vi "Auto - Values into Cluster (SubVI).vi"(6 "Auto Array":dbl[][](array[numeric]), 7 "Was Disabled":bool, 8 "Constant cluster In":T2, 9 "Auton Input Cluster in":T3, 10 "Sensors In":T1, 11 "Auton State":i32) -> (0 "Sensor TypeDef.ctlConstant cluster Out":T2, 1 "Auton Input Cluster With Data":T3, 2 "Sensors Out":T1, 3 "Auton State Out":i32)   [LabVIEW 2020]
uses:
  TypeDefs/Auton Cluster Typedef.ctl
  Disabled/Constant VI_s/Disabled - Constant Cluster Typedef.ctl
  TypeDefs/Sensor TypeDef.ctl
panel:
  # "Controls"
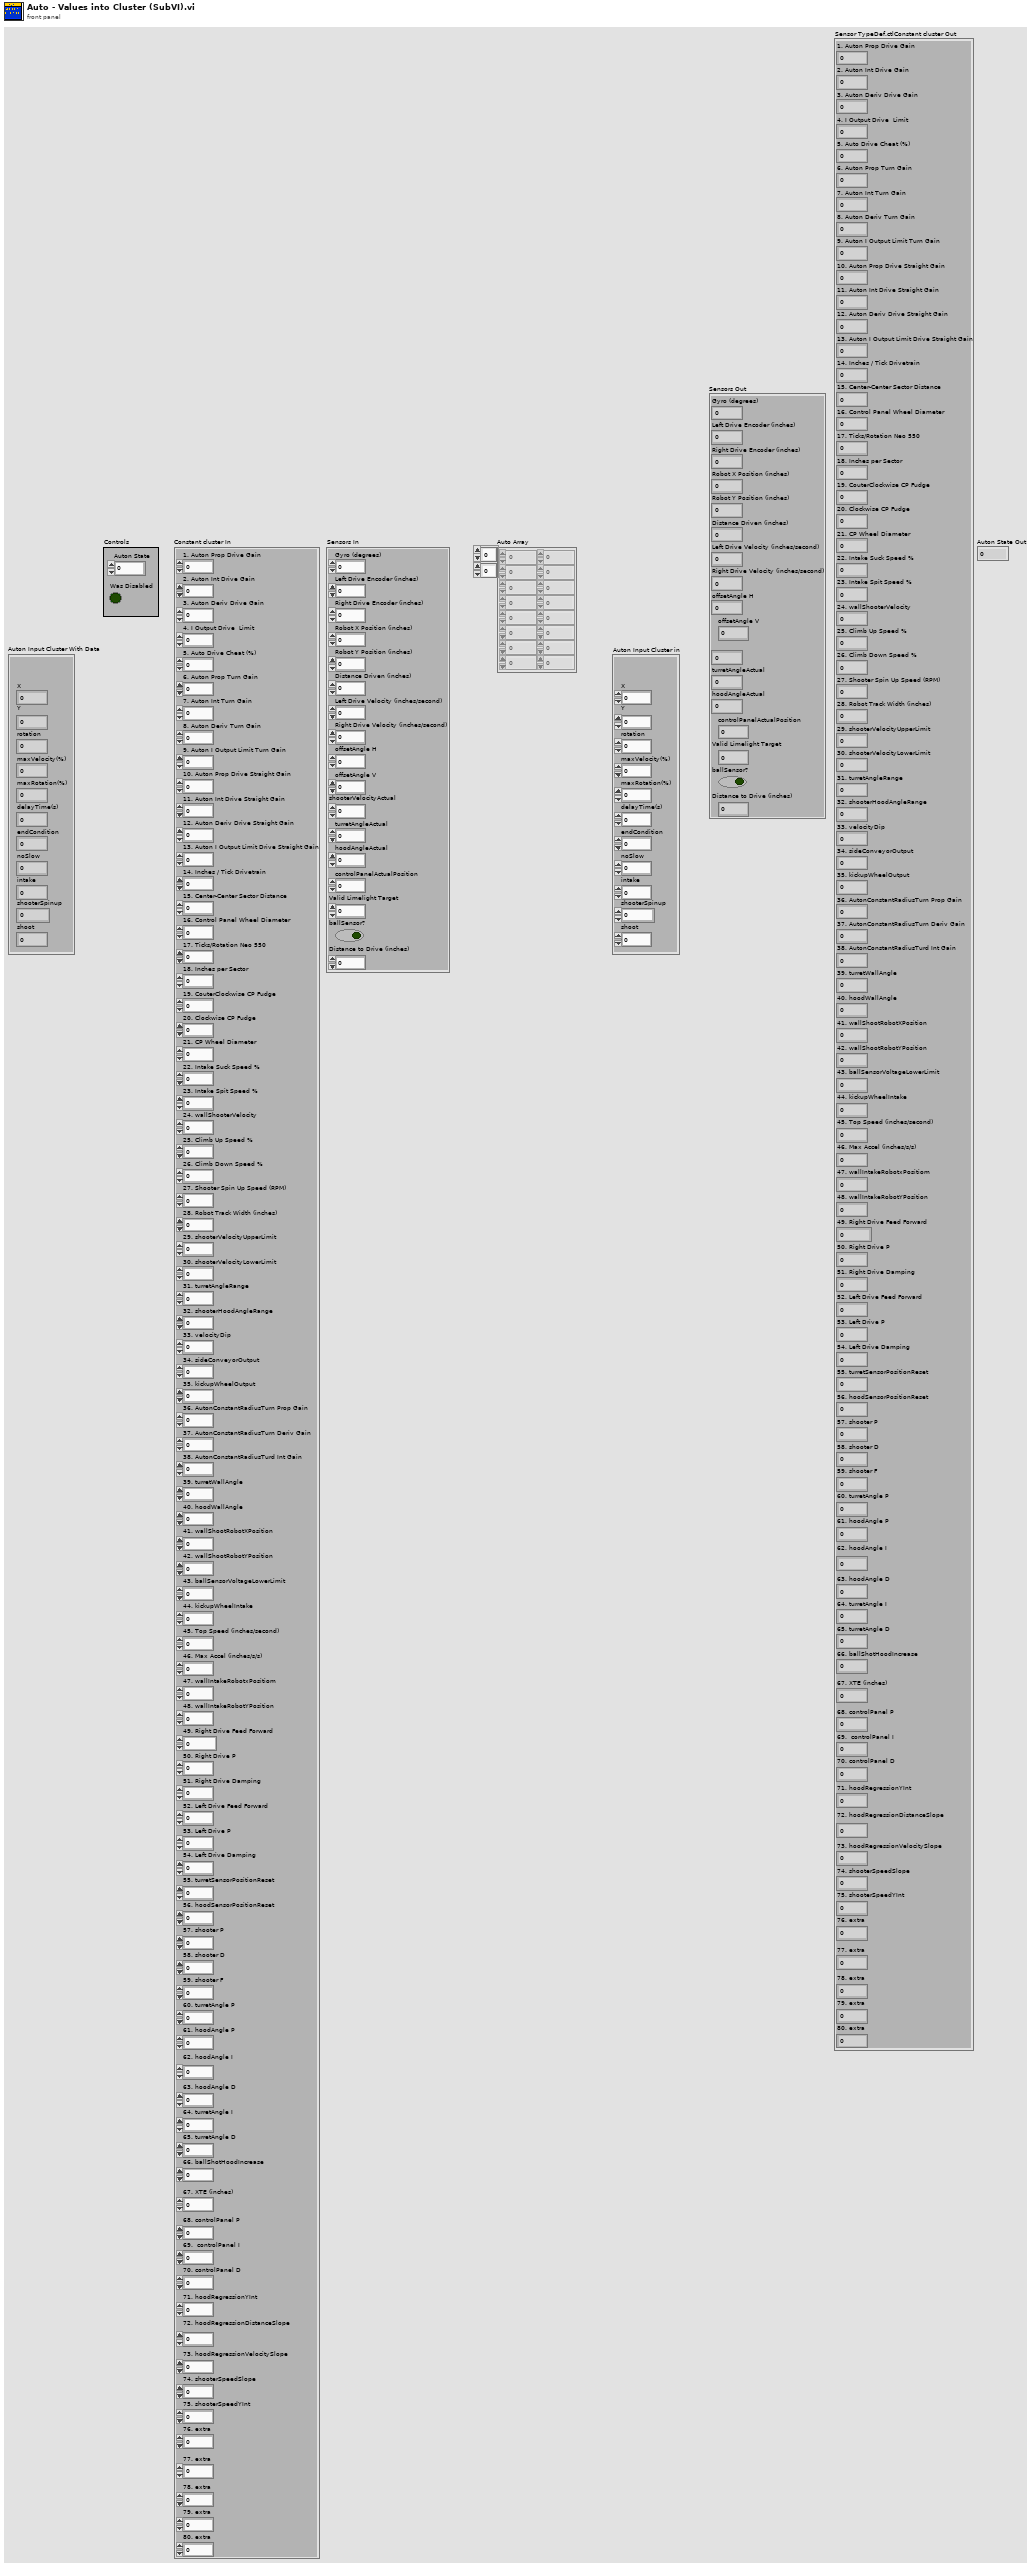
[diagram p1: front panel]
types:
  T1 = typedef "Sensor TypeDef.ctl" = cluster{"Gyro (degrees)":dbl, "Left Drive Encoder (inches)":dbl, "Right Drive Encoder (inches)":dbl, "Robot X Position (inches)":dbl, "Robot Y Position (inches)":dbl, "Distance Driven (inches)":dbl, "Left Drive Velocity (inches/second)":dbl, "Right Drive Velocity (inches/second)":dbl, "offsetAngle H":dbl, "offsetAngle V":dbl, "shooterVelocityActual":dbl, "turretAngleActual":dbl, "hoodAngleActual":dbl, "controlPanelActualPosition":dbl, "Valid Limelight Target":dbl, "ballSensor?":bool, "Distance to Drive (inches)":dbl}
  T2 = typedef "Disabled - Constant Cluster Typedef.ctl" = cluster{"1. Auton Prop Drive Gain":dbl, "2. Auton Int Drive Gain":dbl, "3. Auton Deriv Drive Gain":dbl, "4. I Output Drive  Limit":dbl, "5. Auto Drive Cheat (%)":dbl, "6. Auton Prop Turn Gain":dbl, "7. Auton Int Turn Gain":dbl, "8. Auton Deriv Turn Gain":dbl, "9. Auton I Output Limit Turn Gain":dbl, "10. Auton Prop Drive Straight Gain":dbl, "11. Auton Int Drive Straight Gain":dbl, "12. Auton Deriv Drive Straight Gain":dbl, "13. Auton I Output Limit Drive Straight Gain":dbl, "14. Inches / Tick Drivetrain":dbl, "15. Center-Center Sector Distance":dbl, "16. Control Panel Wheel Diameter":dbl, "17. Ticks/Rotation Neo 550":dbl, "18. Inches per Sector":dbl, "19. CouterClockwise CP Fudge":dbl, "20. Clockwise CP Fudge":dbl, "21. CP Wheel Diameter":dbl, "22. Intake Suck Speed %":dbl, "23. Intake Spit Speed %":dbl, "24. wallShooterVelocity":dbl, "25. Climb Up Speed %":dbl, "26. Climb Down Speed %":dbl, "27. Shooter Spin Up Speed (RPM)":dbl, "28. Robot Track Width (inches)":dbl, "29. shooterVelocityUpperLimit":dbl, "30. shooterVelocityLowerLimit":dbl, "31. turretAngleRange":dbl, "32. shooterHoodAngleRange":dbl, "33. velocityDip":dbl, "34. sideConveyorOutput":dbl, "35. kickupWheelOutput":dbl, "36. AutonConstantRadiusTurn Prop Gain":dbl, "37. AutonConstantRadiusTurn Deriv Gain":dbl, "38. AutonConstantRadiusTurd Int Gain":dbl, "39. turretWallAngle":dbl, "40. hoodWallAngle":dbl, "41. wallShootRobotXPosition":dbl, "42. wallShootRobotYPosition":dbl, "43. ballSensorVoltageLowerLimit":dbl, "44. kickupWheelIntake":dbl, "45. Top Speed (inches/second)":dbl, "46. Max Accel (inches/s/s)":dbl, "47. wallIntakeRobotxPositiom":dbl, "48. wallIntakeRobotYPosition":dbl, "49. Right Drive Feed Forward":dbl, "50. Right Drive P":dbl, "51. Right Drive Damping":dbl, "52. Left Drive Feed Forward":dbl, "53. Left Drive P":dbl, "54. Left Drive Damping":dbl, "55. turretSensorPositionReset":dbl, "56. hoodSensorPositionReset":dbl, "57. shooter P":dbl, "58. shooter D":dbl, "59. shooter F":dbl, "60. turretAngle P":dbl, "61. hoodAngle P":dbl, "62. hoodAngle I":dbl, "63. hoodAngle D":dbl, "64. turretAngle I":dbl, "65. turretAngle D":dbl, "66. ballShotHoodIncrease":dbl, "67. XTE (inches)":dbl, "68. controlPanel P":dbl, "69.  controlPanel I":dbl, "70. controlPanel D":dbl, "71. hoodRegressionYInt":dbl, "72. hoodRegressionDistanceSlope":dbl, "73. hoodRegressionVelocitySlope":dbl, "74. shooterSpeedSlope":dbl, "75. shooterSpeedYInt":dbl, "76. extra":dbl, "77. extra":dbl, "78. extra":dbl, "79. extra":dbl, "80. extra":dbl}
  T3 = typedef "Auton Cluster Typedef.ctl" = cluster{"rotation":dbl, "maxVelocity(%)":dbl, "delayTime(s)":dbl, "endCondition":dbl, "noSlow":dbl, "intake":dbl, "shooterSpinup":dbl, "shoot":dbl, "X":dbl, "Y":dbl, "maxRotation(%)":dbl}
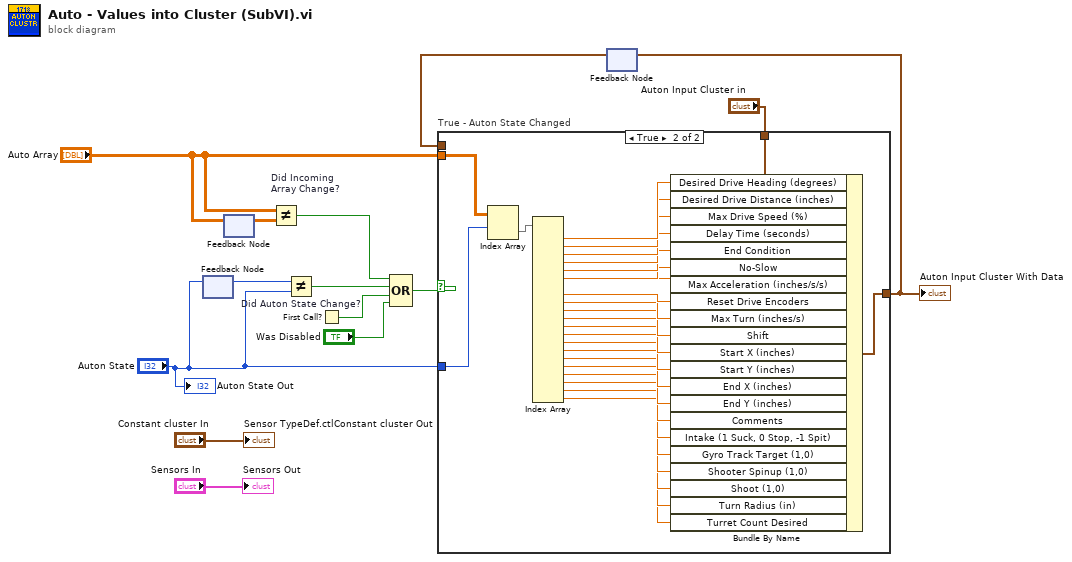
[diagram p0: block diagram]
diagram:
  n1 = feedback-in #1("Auton State") -> ()
  n2 = feedback #1() -> (w2:i32)  [unwired: 1 in]
  n3 = feedback #2() -> (w11:dbl[][])  [unwired: 1 in]
  n4 = feedback-in #2("Auto Array") -> ()
  n5 = Not Equal? "Did Incoming\nArray Change?"(x="Auto Array", y=w11) -> (x != y?=w7:bool)
  n6 = Not Equal? "Did Auton State Change?"(x=w2, y="Auton State") -> (x != y?=w10:bool)
  n7 = First Call?() -> (First Call?: T/F=w9:bool)
  n8 = Compound Arithmetic op=OR(w7, w10, w9, "Was Disabled") -> (w8:bool)
  n9 = feedback #3() -> (w12:T3)  [unwired: 1 in]
  n10 = case "True - Auton State Changed" shown="True" w8 {
    tunnel: [w15 w41] -> w13
    tunnel: "Auton Input Cluster in" -> [_ w40]
    tunnel: "Auton State" -> [_ w39]
    tunnel: w12 -> [w15 _]
    tunnel: "Auto Array" -> [_ w38]
    frame False {
    }
    frame True {
      n11 = Index Array(array=w38, index (row)=w39) -> (element=w37:dbl[])  [unwired: 1 in]
      n12 = Index Array(array=w37) -> (element #1=w36:dbl, element #2=w35:dbl, element #3=w34:dbl, element #4=w33:dbl, element #5=w32:dbl, element #6=w31:dbl, element #7=w30:dbl, element #8=w29:dbl, element #9=w28:dbl, element #10=w27:dbl, element #11=w26:dbl, element #12=w25:dbl, element #13=w24:dbl, element #14=w23:dbl, element #15=w22:dbl, element #16=w21:dbl, element #17=w20:dbl, element #18=w19:dbl, element #19=w18:dbl, element #20=w17:dbl, element #21=w16:dbl)  [unwired: 21 in]
      n13 = Bundle By Name(cluster=w40, "Desired Drive Heading (degrees)"=w36, "Desired Drive Distance (inches)"=w35, "Max Drive Speed (%)"=w34, "Delay Time (seconds)"=w33, "End Condition"=w32, "No-Slow"=w31, "Max Acceleration (inches/s/s)"=w30, "Reset Drive Encoders"=w29, "Max Turn (inches/s)"=w28, "Shift"=w27, "Start X (inches)"=w26, "Start Y (inches)"=w25, "End X (inches)"=w24, "End Y (inches)"=w23, "Comments"=w22, "Intake (1 Suck, 0 Stop, -1 Spit)"=w21, "Gyro Track Target (1,0)"=w20, "Shooter Spinup (1,0)"=w19, "Shoot (1,0)"=w18, "Turn Radius (in)"=w17, "Turret Count Desired"=w16) -> (w41:T3)
    }
  }
  "Auton Input Cluster With Data" <- w13
  n14 = feedback-in #3(w13) -> ()
  "Sensor TypeDef.ctlConstant cluster Out" <- "Constant cluster In"
  "Sensors Out" <- "Sensors In"
  "Auton State Out" <- "Auton State"
